vi "FGV_Cards.vi"(7 "Action":T3=enum."Set_VCHCards", 10 "error in (no error)":errorcluster caption="错误输入（无错误）", 11 "Cards in":T1[](array[typedef])) -> (2 "error out":errorcluster caption="错误输出", 3 "Cards out":T1[](array[typedef]))   [LabVIEW 2016]
uses:
  FGV_Cards.ctl
  Controls/PSCHN_Card Para.ctl
  Controls/PSCHN_Channel Para.ctl
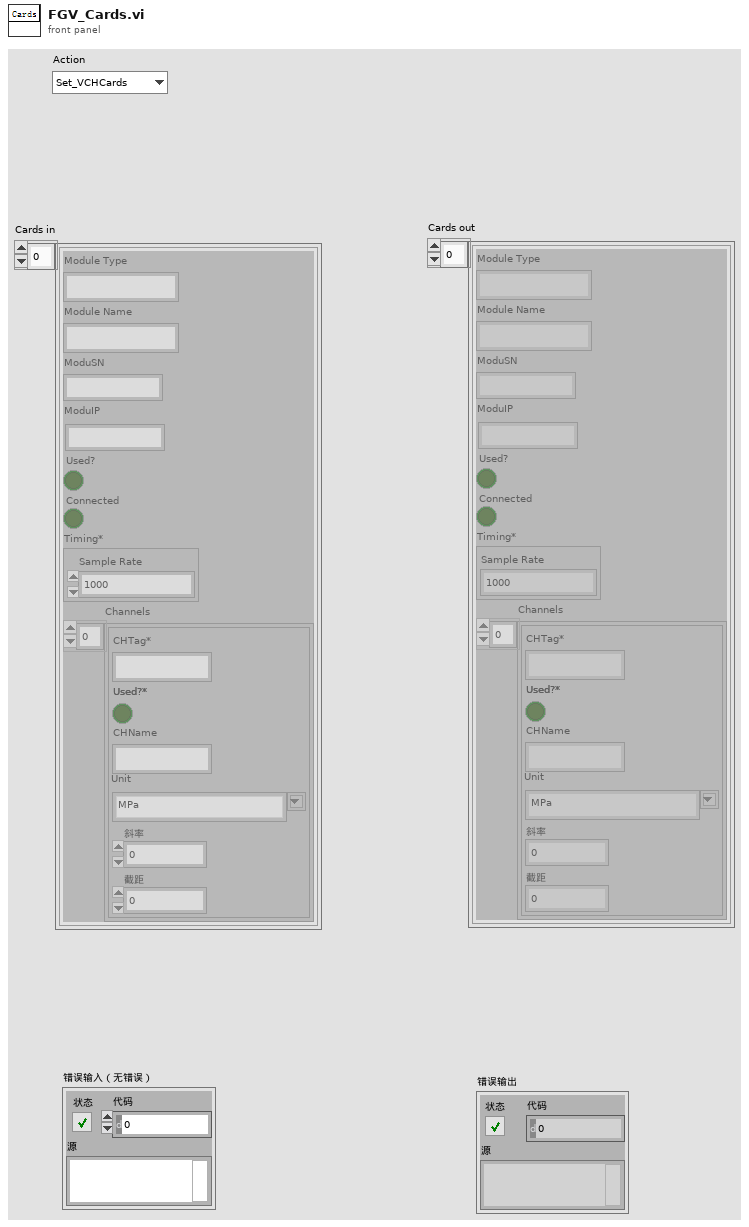
[diagram p1: front panel]
types:
  T1 = typedef "PSCHN_Card Para.ctl" = cluster{"Module Type":string, "Module Name":string, "ModuSN":string, "ModuIP":string, "Used?":bool, "Connected":bool, "Timing*":cluster{"Sample Rate":dbl}, "Channels":T2[]}
  T2 = typedef "PSCHN_Channel Para.ctl" = cluster{"CHTag*":string, "Used?*":bool, "CHName":string, "Unit":string, "斜率":dbl, "截距":dbl}
  T3 = typedef "FGV_Cards.ctl" = enum16{"Initlize", "Set_DAQCards", "Set_VCHCards", "Get_DAQCards", "Get_VCHCards", "Get_ALLUsing"}
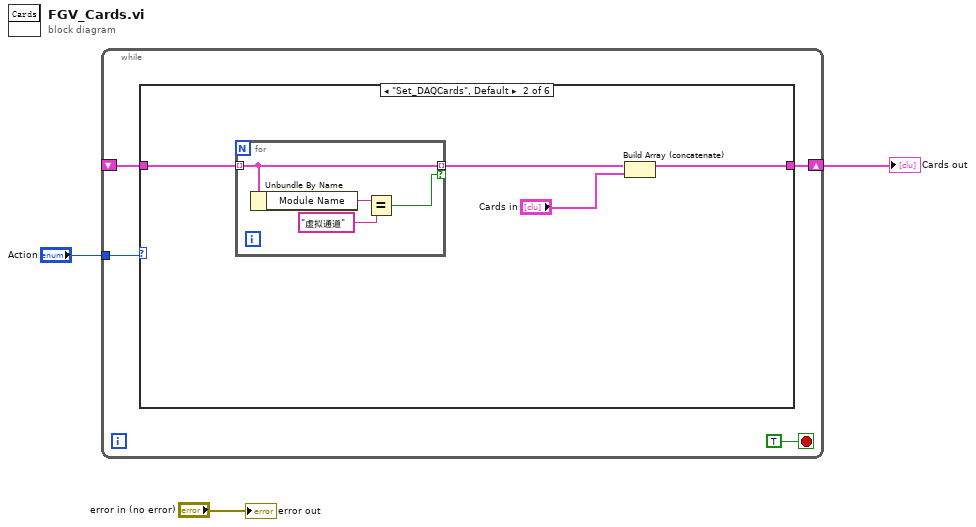
[diagram p0: block diagram]
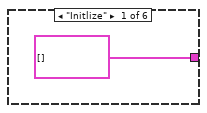
[diagram p2: hidden frame]
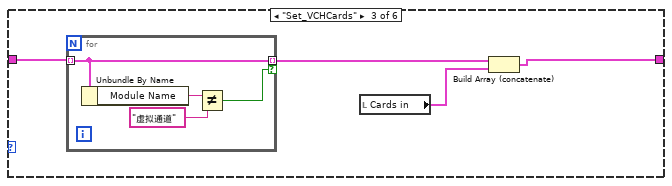
[diagram p3: hidden frame]
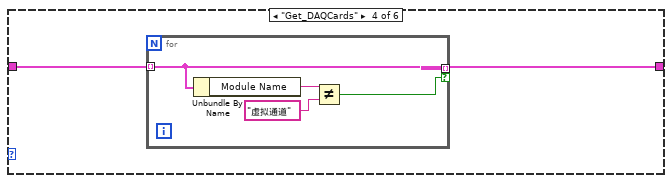
[diagram p4: hidden frame]
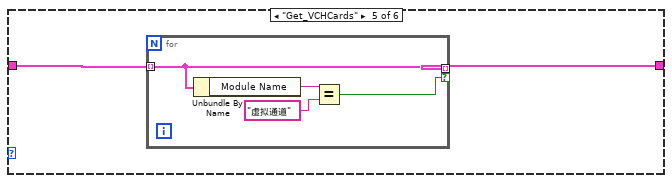
[diagram p5: hidden frame]
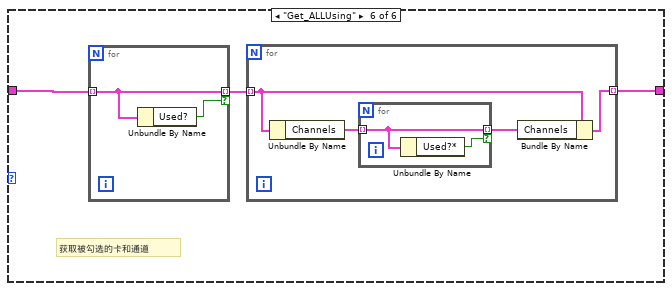
[diagram p6: hidden frame]
diagram:
  n1 = while {
    tunnel: "Action" -> [w6]
    shift-right: [w5] -> w1
    shift-left: _ -> [w4]
    stop <- TRUE stop-if-true
    n2 = case shown="\"Set_DAQCards\", Default" w6 {
      tunnel: [T1[] [] ("Cards in") w11 w19 w25 w31 w37] -> w5
      tunnel: w4 -> [_ w10 w18 w26 w32 w39]
      frame "Initlize" {
      }
      frame "Set_DAQCards", Default {
        n3 = for {
          tunnel: w10 -> [w14] mode=indexing
          tunnel: [w14] -> w9 mode=indexing if=w13
          n4 = Unbundle By Name(w14) -> ("Module Name"=w16:string)
          n5 = Equal?(x=w16, y="虚拟通道") -> (x = y?=w13:bool)
        }
        n6 = Build Array (concatenate)(w9, "Cards in") -> (w11:T1[])
      }
      frame "Set_VCHCards" {
        n7 = for {
          tunnel: w18 -> [w22] mode=indexing
          tunnel: [w22] -> w17 mode=indexing if=w21
          n8 = Unbundle By Name(w22) -> ("Module Name"=w24:string)
          n9 = Not Equal?(x=w24, y="虚拟通道") -> (x != y?=w21:bool)
        }
        n10 = local read "Cards in"() -> (w20:T1[])
        n11 = Build Array (concatenate)(w17, w20) -> (w19:T1[])
      }
      frame "Get_DAQCards" {
        n12 = for {
          tunnel: w26 -> [w29] mode=indexing
          tunnel: [w29] -> w25 mode=indexing if=w27
          n13 = Unbundle By Name(w29) -> ("Module Name"=w30:string)
          n14 = Not Equal?(x=w30, y="虚拟通道") -> (x != y?=w27:bool)
        }
      }
      frame "Get_VCHCards" {
        n15 = for {
          tunnel: w32 -> [w35] mode=indexing
          tunnel: [w35] -> w31 mode=indexing if=w33
          n16 = Unbundle By Name(w35) -> ("Module Name"=w36:string)
          n17 = Equal?(x=w36, y="虚拟通道") -> (x = y?=w33:bool)
        }
      }
      frame "Get_ALLUsing" {
        # "获取被勾选的卡和通道"
        n18 = for {
          tunnel: w39 -> [w47] mode=indexing
          tunnel: [w47] -> w38 mode=indexing if=w46
          n19 = Unbundle By Name(w47) -> ("Used?"=w46:bool)
        }
        n20 = for {
          tunnel: w38 -> [w42] mode=indexing
          tunnel: [w40] -> w37 mode=indexing
          n21 = Unbundle By Name(w42) -> ("Channels"=w43:T2[])
          n22 = for {
            tunnel: w43 -> [w45] mode=indexing
            tunnel: [w45] -> w41 mode=indexing if=w44
            n23 = Unbundle By Name(w45) -> ("Used?*"=w44:bool)
          }
          n24 = Bundle By Name(cluster=w42, "Channels"=w41) -> (w40:T1)
        }
      }
    }
  }
  "Cards out" <- w1
  "error out" <- "error in (no error)"
